vi "tb_logabsmag.vi"() -> ()   [LabVIEW 2011]
uses:
  <vilib>/rvi/XilinxIP/XIPIN_XNode/niFpgaXIPIN.xnode
  <userlib>/FPGA Library/Code Development/Signal Processing/FFT Block/Logarithm/Temp/tb_logabsmag/fxptosgl/fxptosgl_C37418154DA4454766780DA4BC935102.dll
  <vilib>/rvi/IPIntegrationNode/IPINode_Xnode/niFpgaIPINode.xnode
  <vilib>/rvi/IPIntegrationNode/IPINode_Utilities/niFpgaIPINodeSimCore.vi
  <userlib>/FPGA Library/Code Development/Signal Processing/FFT Block/Logarithm/Temp/tb_logabsmag/sqrfloat/sqrfloat_3DE220F74732280EA0AECCBEDDA90502.dll
  <userlib>/FPGA Library/Code Development/Signal Processing/FFT Block/Logarithm/Temp/tb_logabsmag/SGLAdd/SGLAdd_37168F5440D705665131A18EEC9F8D92.dll
panel:
  out "error":dbl
  out "x+y":dbl
  out "Output":dbl
  out "Exponent":fxp<+/-,9,9>
  out "FXP Part":fxp<+/-,25,2> format="%.25g"
  in  "y":fxp<+/-,32,1> format="%.6f"
  in  "x":fxp<+/-,32,1> format="%.6f"
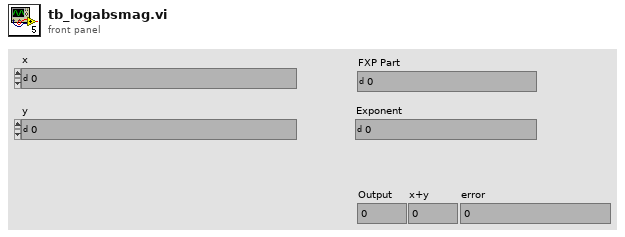
[diagram p1: front panel]
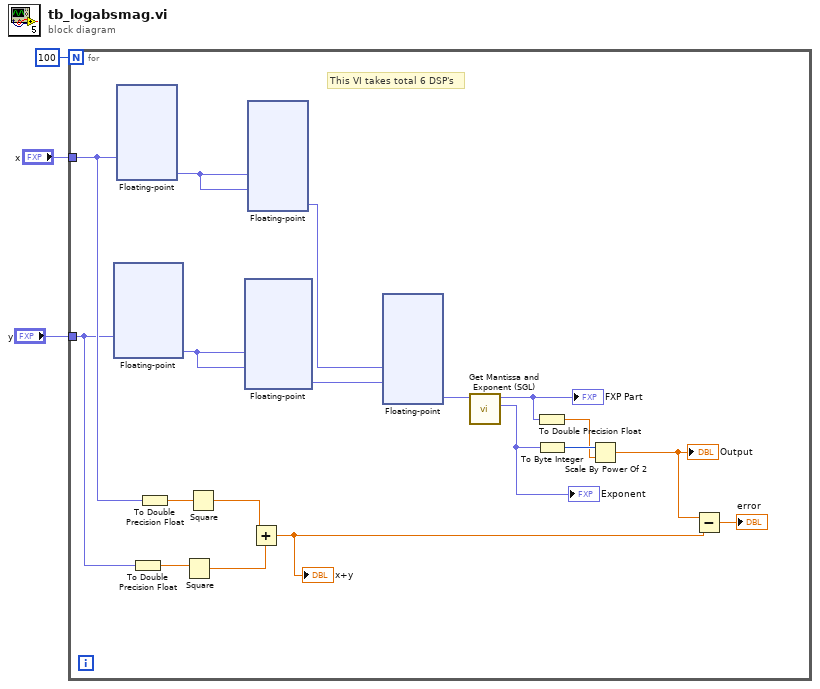
[diagram p0: block diagram]
diagram:
  n1 = for {
    N: 100 -> [_]
    tunnel: "x" -> [w12]
    tunnel: "y" -> [w11]
    # "This VI takes total 6 DSP's"
    n2 = xnode ("Floating-point")("a"=w11) -> ("result"=w19:fxp<+/-,32,32>)
    n3 = xnode ("Floating-point")("a"=w12) -> ("result"=w21:fxp<+/-,32,32>)
    n4 = To Double Precision Float(number=w11) -> (double precision float=w9:dbl)
    n5 = To Double Precision Float(number=w12) -> (double precision float=w10:dbl)
    n6 = Square(x=w9) -> (x^2=w7:dbl)
    n7 = Square(x=w10) -> (x^2=w8:dbl)
    n8 = xnode ("Floating-point")("a"=w19, "b"=w19) -> ("result"=w18:fxp<+/-,32,32>)
    n9 = xnode ("Floating-point")("a"=w21, "b"=w21) -> ("result"=w20:fxp<+/-,32,32>)
    n10 = Add(x=w8, y=w7) -> (x+y=w5:dbl)
    "x+y" <- w5
    n11 = xnode ("Floating-point")("a"=w20, "b"=w18) -> ("result"=w17:fxp<+/-,32,32>)
    n12 = call <userlib>:"Get Mantissa and Exponent (SGL).vi"("Input"=w17) -> ("Exponent"=w15:fxp<+/-,9,9>, "FXP Part"=w16:fxp<+/-,25,2>)  [unwired: 9 in]
    "FXP Part" <- w16
    "Exponent" <- w15
    n13 = To Double Precision Float(number=w16) -> (double precision float=w13:dbl)
    n14 = To Byte Integer(number=w15) -> (8bit integer=w14:i8)
    n15 = Scale By Power Of 2(n=w14, x=w13) -> (x*2^n=w6:dbl)
    "Output" <- w6
    n16 = Subtract(x=w6, y=w5) -> (x-y=→"error":dbl)
  }
